vi "Parse Structure Recursive.vi"(8 "error in":errorcluster, 10 "Structure In":refnum<class "Tree.lvclass">, 11 "Tree In":refnum<class "Tree.lvclass">) -> (0 "error out":errorcluster, 1 "Geometric":refnum<class "Geometric.lvclass">[](array[class]), 2 "Structure Out":refnum<class "Tree.lvclass">, 3 "Tree Out":refnum<class "Tree.lvclass">)   [LabVIEW 2019, in "ParseGDSII.lvclass"]
uses:
  ParseGDSII.lvclass
  Tree/Tree.lvclass
  Elements/Geometric.lvclass
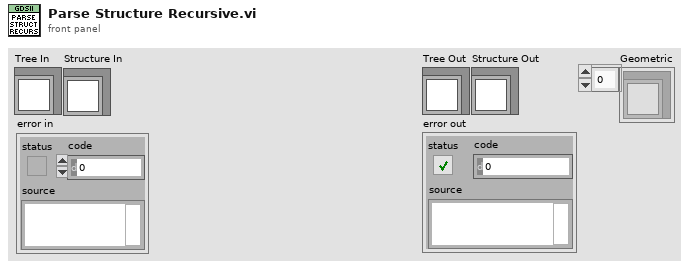
[diagram p1: front panel]
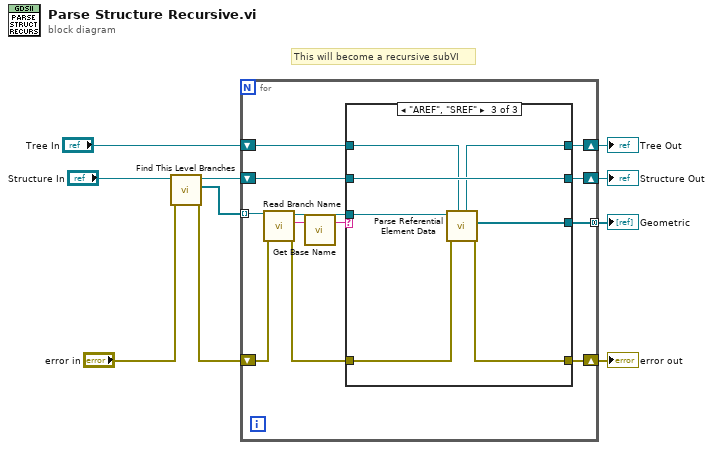
[diagram p0: block diagram]
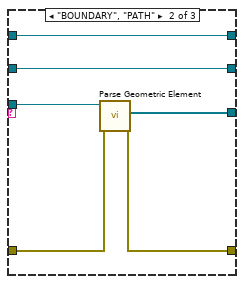
[diagram p3: hidden frame]
diagram:
  # "This will become a recursive subVI"
  n1 = call "Find This Level Branches.vi"("error in"="error in", "Tree in"="Structure In") -> ("error out"=w8:errorcluster, "Branches"=w10:refnum<class "Tree.lvclass">[], "Tree out"=w9:refnum<class "Tree.lvclass">)  [unwired: 7 in]
  n2 = for {
    shift-right: [w15] -> w4
    shift-left: "Tree In" -> [w17]
    tunnel: w10 -> [w22] mode=indexing
    shift-right: [w16] -> w3
    shift-left: w9 -> [w18]
    shift-right: [w12] -> w2
    shift-left: w8 -> [w20]
    tunnel: [w11] -> w1 mode=concatenating
    n3 = call "Read Branch Name.vi"("error in"=w20, "Tree in"=w22) -> ("error out"=w13:errorcluster, "Branch Name"=w21:string, "Tree out"=w14:refnum<class "Tree.lvclass">)  [unwired: 7 in]
    n4 = call "Get Base Name.vi"("Unique Name"=w21) -> ("Base Name"=w19:string)  [unwired: 2 in]
    n5 = case shown="\"AREF\", \"SREF\"" w19 {
      tunnel: w18 -> [w25 w31 w38]
      tunnel: w17 -> [w24 w30 w35]
      tunnel: [w25 w31 w38] -> w16
      tunnel: [w24 w30 w36] -> w15
      tunnel: w14 -> [_ w29 w37]
      tunnel: w13 -> [w23 w27 w32]
      tunnel: [w23 w28 w33] -> w12
      tunnel: [_ w26 w34] -> w11
      frame Default {
      }
      frame "BOUNDARY", "PATH" {
        n6 = call "Parse Geometric Element.vi"("error in"=w27, "Element In"=w29) -> ("error out"=w28:errorcluster, "Geometric"=w26:refnum<class "Geometric.lvclass">[])  [unwired: 7 in, 1 out]
      }
      frame "AREF", "SREF" {
        n7 = call "Parse Referential Element Data.vi"("Tree In"=w35, "error in"=w32, "Element In"=w37) -> ("error out"=w33:errorcluster, "Geometric"=w34:refnum<class "Geometric.lvclass">[], "Tree Out"=w36:refnum<class "Tree.lvclass">)  [unwired: 5 in, 1 out]
      }
    }
  }
  "Tree Out" <- w4
  "Structure Out" <- w3
  "error out" <- w2
  "Geometric" <- w1
